vi "Global_time(SubVI).vi"(11 "R/W":enum16{"Write", "Read", "RAZ"}(ring)) -> (2 "D_time":u32)   [LabVIEW 2015]
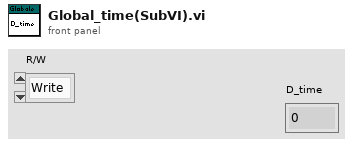
[diagram p1: front panel]
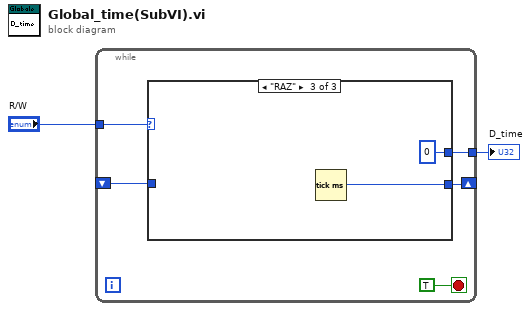
[diagram p0: block diagram]
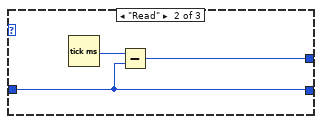
[diagram p3: hidden frame]
diagram:
  n1 = while {
    tunnel: "R/W" -> [w7]
    shift-right: [w5] -> _
    shift-left: _ -> [w4]
    tunnel: [w3] -> w1
    stop <- TRUE stop-if-true
    n2 = case shown="\"RAZ\"" w7 {
      tunnel: [w8 w10 w13] -> w5
      tunnel: w4 -> [w8 w10 _]
      tunnel: [_ w9 u32 0] -> w3
      frame "Write", Default {
      }
      frame "Read" {
        n3 = Tick Count (ms)() -> (millisecond timer value=w11:u32)
        n4 = Subtract(x=w11, y=w10) -> (x-y=w9:u32)
      }
      frame "RAZ" {
        n5 = Tick Count (ms)() -> (millisecond timer value=w13:u32)
      }
    }
  }
  "D_time" <- w1
